vi "setUp.vi"(8 "error in":errorcluster, 11 "reference in":refnum<class "Create Execution Unit.lvclass">) -> (0 "error out":errorcluster, 3 "reference out":refnum<class "Create Execution Unit.lvclass">)   [LabVIEW 2020, in "Create Execution Unit.lvclass"]
doc: "setUp runs prior to the test method during test execution. Use this method to initialize any object data required by your tests."
uses:
  Create Execution Unit.lvclass
  C:/dev/git/niveristand-custom-device-testing-tools/VeriStandScriptingTestCase/VeriStandScriptingTestCase.lvclass
  C:/Program Files (x86)/National Instruments/LabVIEW 2020/vi.lib/addons/_JKI Toolkits/VI Tester/TestCase.llb/TestCase.lvclass
  Create Execution Unit.lvclass/Create Execution Unit.ctl
  Hardware API/Global - Disable Hardware API Constant.vi
  <vilib>/addons/_JKI Toolkits/VI Tester/TestCase.llb/TestCase.lvclass
  niveristand-custom-device-testing-tools/VeriStandScriptingTestCase/VeriStandScriptingTestCase.lvclass
  niveristand-custom-device-testing-tools/VeriStandTestUtilities/VeriStandTestUtilities.lvlib
  Hardware API/AIM MIL-STD-1553 Hardware API.lvlib
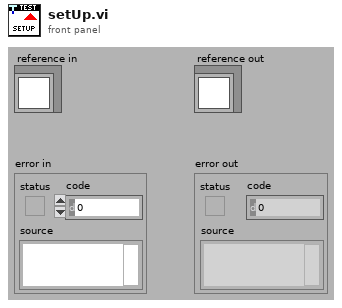
[diagram p1: front panel]
types:
  T1 = enum16{"Enabled (Default)", "Disabled for Unit Testing"}
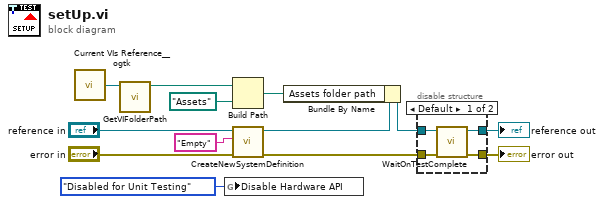
[diagram p0: block diagram]
diagram:
  n1 = call <userlib>:"Current VIs Reference__ogtk.vi"() -> ("Current VI's reference"=w7:refnum<vi>)  [unwired: 5 in]
  n2 = call "GetVIFolderPath.vi"("VI Reference in"=w7) -> ("VI Folder Path out"=w6:path)  [unwired: 9 in, 1 out]
  n3 = global write "Global - Disable Hardware API Constant.vi" "Disable Hardware API"(T1."Disabled for Unit Testing" ("Disable Hardware API")) -> ()
  n4 = Build Path(base path=w6, name or relative path=path "Assets") -> (appended path=w4:path)
  n5 = call "CreateNewSystemDefinition.vi"("error in (no error)"="error in", "System Definition Name"="Empty", "VeriStandScriptingTestCase in"="reference in") -> ("error out"=w8:errorcluster, "VeriStandScriptingTestCase out"=w3:refnum<class "Create Execution Unit.lvclass">)  [unwired: 7 in]
  n6 = Bundle By Name(cluster=w3, "Assets folder path"=w4) -> (w2:refnum<class "Create Execution Unit.lvclass">)
  n7 = disable-structure shown="Default" {
    disable-tunnel: w8 -> [w17 w18]
    disable-tunnel: [w16 w18] -> w13
    disable-tunnel: [w15 w19] -> w12
    disable-tunnel: w2 -> [w14 w19]
    frame condition #0 (active) {
      n8 = call <vilib>:"WaitOnTestComplete.vi"("error in (no error)"=w17, "TestCase in"=w14) -> ("error out"=w16:errorcluster, "TestCase out"=w15:refnum<class "Create Execution Unit.lvclass">)  [unwired: 8 in]
    }
    frame condition #1 {
    }
  }
  "error out" <- w13
  "reference out" <- w12
